vi "get display name.vi"(8 "error in":errorcluster, 11 "set source separate in":refnum<class "set source separate.lvclass">) -> (0 "error out":errorcluster, 2 "class name":string, 3 "set source separate out":refnum<class "set source separate.lvclass">)   [LabVIEW 2013, in "set source separate.lvclass"]
uses:
  set source separate.lvclass
  VI modification.lvclass
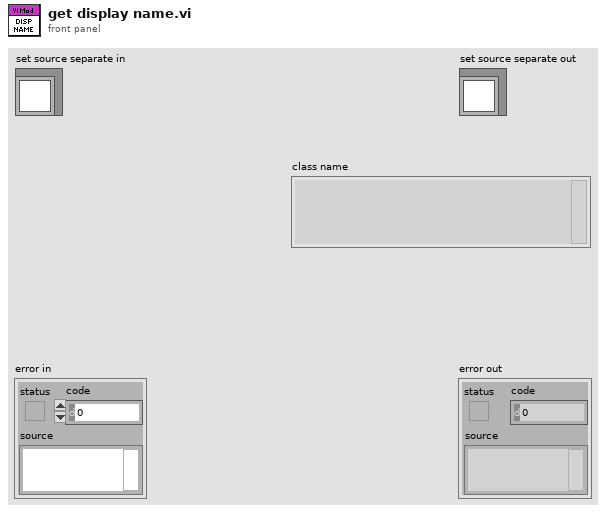
[diagram p1: front panel]
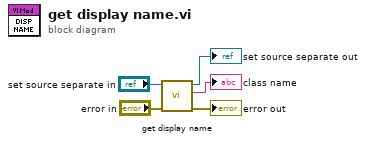
[diagram p0: block diagram]
diagram:
  n1 = call-parent "get display name.vi"("error in"="error in", "VI modification in"="set source separate in") -> ("error out"=→"error out":errorcluster, "class name"=→"class name":string, "VI modification out"=→"set source separate out":refnum<class "set source separate.lvclass">)  [unwired: 7 in]
